vi "toml_file_remove.vi"(8 "error in (no error)":errorcluster, 10 "delete file on disk? (F)":bool, 11 "path in":path) -> (0 "error out":errorcluster, 3 "path out":path)   [LabVIEW 2017]
uses:
  toml_fg_action.ctl
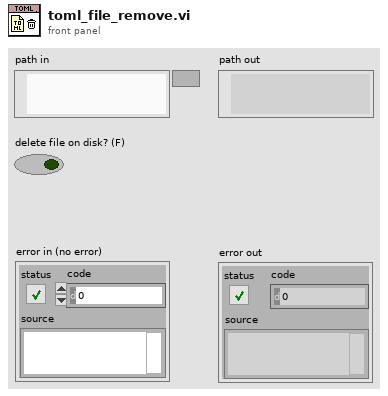
[diagram p1: front panel]
types:
  T1 = typedef "toml_fg_action.ctl" = enum8{"null", "get", "set", "pop", "import", "export", "drop", "sections", "keys", "remove"}
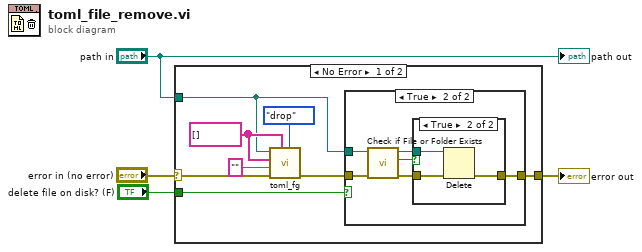
[diagram p0: block diagram]
diagram:
  n1 = case shown="No Error" "error in (no error)" {
    selector: "error in (no error)" -> [w12 w24]
    tunnel: [w6 w24] -> w3
    tunnel: "path in" -> [w7 _]
    tunnel: "delete file on disk? (F)" -> [w5 _]
    frame No Error {
      w10 = string[] [] ("section")
      n2 = call "toml_fg.vi"("action"=toml_fg_action."drop", "section"=w10, "error in (no error)"=w12, "value in"="", "key"=w10, "path in"=w7) -> ("error out"=w8:errorcluster)  [unwired: 2 in, 3 out]
      n3 = case shown="True" w5 {
        tunnel: w8 -> [w13 w19]
        tunnel: w7 -> [_ w18]
        tunnel: [w13 w16] -> w6
        frame False {
        }
        frame True {
          n4 = call <vilib>:"Check if File or Folder Exists.vi"("error in (no error)"=w19, "path"=w18) -> ("error out"=w17:errorcluster, "file or folder exists?"=w14:bool, "dup path"=w15:path)  [unwired: 7 in]
          n5 = case shown="True" w14 {
            tunnel: w17 -> [w20 w23]
            tunnel: [w20 w22] -> w16
            tunnel: w15 -> [_ w21]
            frame False {
            }
            frame True {
              n6 = Delete(path (use dialog)=w21, error in=w23) -> (error out=w22:errorcluster)  [unwired: 3 in, 2 out]
            }
          }
        }
      }
    }
    frame Error {
    }
  }
  "error out" <- w3
  "path out" <- "path in"
